vi "Mov_Avg_JS.vi"(8 "Array In":dbl[](array[numeric]), 9 "Cycle Length":dbl, 10 "Input":dbl) -> (0 "Array Out Main":dbl[](array[numeric]), 2 "Mean":dbl format="%0.2f")   [LabVIEW 2014]
uses:
  <vilib>/Analysis/baseanly.llb/Mean (DBL).vi
  <vilib>/Analysis/NI_AALBase.lvlib
panel:
  # "Moving Average VI"
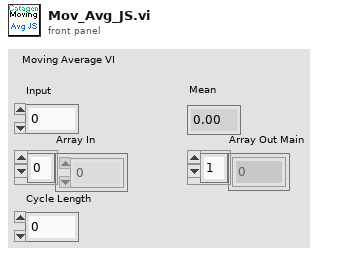
[diagram p1: front panel]
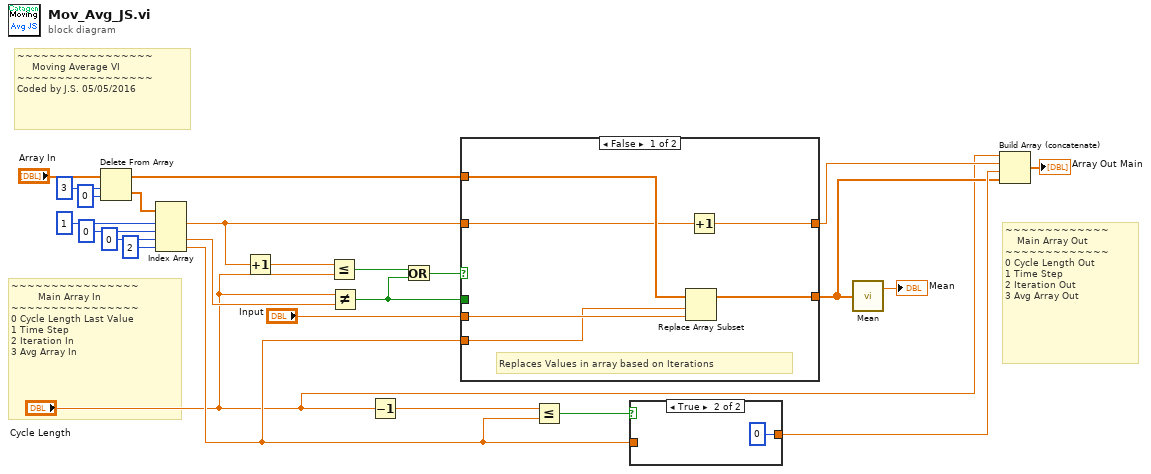
[diagram p0: block diagram]
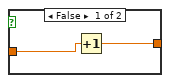
[diagram p2: hidden frame]
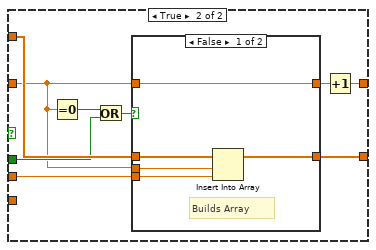
[diagram p3: hidden frame]
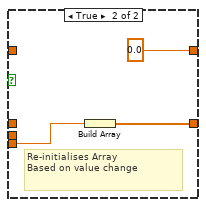
[diagram p4: hidden frame]
diagram:
  # "~~~~~~~~~~~~~~~~\n         Main Array In\n~~~~~~~~~~~~~~~~\n0 Cycle Length Last Value\n1 Time Step\n2 Iteration In\n3 Avg Array In"
  # "~~~~~~~~~~~~~\n    Main Array Out\n~~~~~~~~~~~~~\n0 Cycle Length Out\n1 Time Step\n2 Iteration Out\n3 Avg Array Out"
  # "~~~~~~~~~~~~~~~~~\n     Moving Average VI \n~~~~~~~~~~~~~~~~~\nCoded by J.S. 05/05/2016"
  n1 = Delete From Array(array="Array In", length=3, index=0) -> (deleted portion=w15:dbl[], array with subset deleted=w11:dbl[])
  n2 = Index Array(array=w15, index #1=1 ("index"), index #2=0 ("index"), index #3=0 ("index"), index #4=2 ("index")) -> (element #1=w4:dbl, element #3=w8:dbl, element #4=w6:dbl)  [unwired: 1 out]
  n3 = Increment(x=w4) -> (x+1=w3:dbl)
  n4 = Less Or Equal?(x=w3, y="Cycle Length") -> (x <= y?=w24:bool)
  n5 = Not Equal?(x="Cycle Length", y=w8) -> (x != y?=w22:bool)
  n6 = Decrement(x="Cycle Length") -> (x-1=w20:dbl)
  n7 = Or(x=w24, y=w22) -> (x .or. y?=w25:bool)
  n8 = case shown="False" w25 {
    tunnel: "Input" -> [w29 w39]
    tunnel: [w30 w38] -> w17
    tunnel: w11 -> [w31 w40]
    tunnel: w6 -> [w28 _]
    tunnel: w4 -> [w27 w34]
    tunnel: w22 -> [_ w37]
    tunnel: [w26 w33] -> w2
    frame False {
      # "Replaces Values in array based on Iterations"
      n9 = Replace Array Subset(array=w31, new element=w29, index=w28) -> (w30:dbl[])
      n10 = Increment(x=w27) -> (x+1=w26:dbl)
    }
    frame True {
      n11 = Equal To 0?(x=w34) -> (x = 0?=w35:bool)
      n12 = Or(x=w35, y=w37) -> (x .or. y?=w36:bool)
      n13 = case shown="False" w36 {
        tunnel: w40 -> [w45 _]
        tunnel: w39 -> [w44 w47]
        tunnel: [w43 w48] -> w38
        tunnel: w34 -> [w42 _]
        tunnel: w34 -> [w41 _]
        tunnel: [w41 0.0] -> w32
        frame False {
          # "Builds Array"
          n14 = Insert Into Array(array=w45, index=w42, new element=w44) -> (w43:dbl[])
        }
        frame True {
          # "Re-initialises Array\nBased on value change"
          n15 = Build Array(w47) -> (w48:dbl[])
        }
      }
      n16 = Increment(x=w32) -> (x+1=w33:dbl)
    }
  }
  n17 = Less Or Equal?(x=w20, y=w6) -> (x <= y?=w21:bool)
  n18 = case shown="True" w21 {
    tunnel: [w50 i64 0] -> w18
    tunnel: w6 -> [w49 _]
    frame False {
      n19 = Increment(x=w49) -> (x+1=w50:dbl)
    }
    frame True {
    }
  }
  n20 = call-poly <vilib>:"Mean.vi"("X"=w17) -> ("mean"=→"Mean":dbl)  [unwired: 1 out]
  n21 = Build Array (concatenate)("Cycle Length", w2, w18, w17) -> (→"Array Out Main":dbl[])
